vi "set_CurrentBias.vi"() -> ()   [LabVIEW 2014]
panel:
  out "Dup Aardvark Handle":i32
  out "Data Written":bool
  out "error out":errorcluster
  in  "error in (no error)":errorcluster
  in  "Address (0x50)":u16=80 max=1023 format="%.0x"
  in  "Aardvark Handle":i32 min=0
  in  "Current":dbl
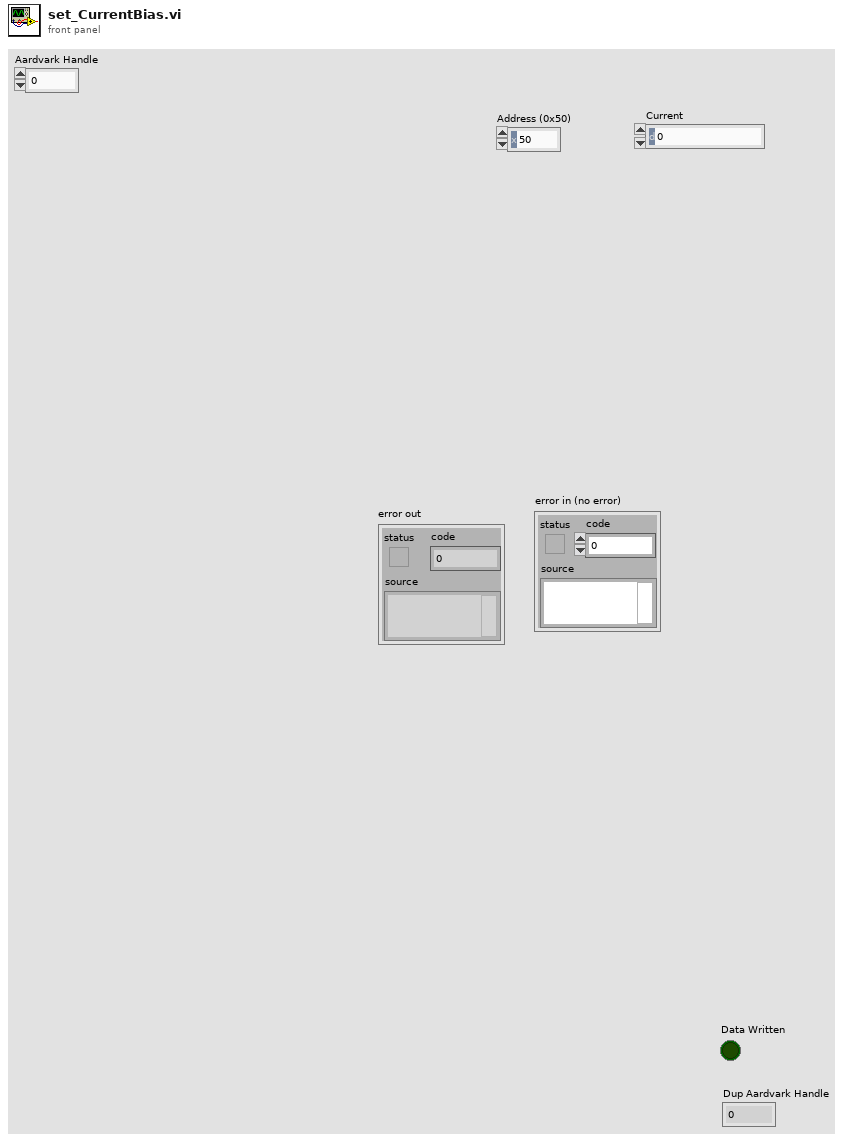
[diagram p1: front panel]
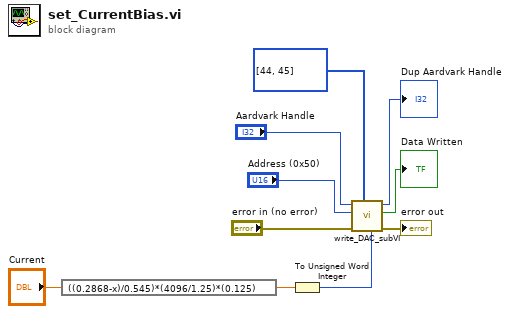
[diagram p0: block diagram]
diagram:
  n1 = expression code="((0.2868-x)/0.545)*(4096/1.25)*(0.125)"("Current") -> (w9:dbl)
  n2 = To Unsigned Word Integer(number=w9) -> (unsigned 16bit integer=w6:u16)
  n3 = call "write_DAC_subVI.vi"("Aardvark Handle in"="Aardvark Handle", "Address (0x50) in"="Address (0x50)", "error in (no error)"="error in (no error)", "DAC_ADD"=u16[] [44, 45], "DAC_Val"=w6) -> ("Dup Aardvark Handle"=→"Dup Aardvark Handle":i32, "DAC Written"=→"Data Written":bool, "error out"=→"error out":errorcluster)  [unwired: 3 in]
